vi "Core.vi"(8 "error in (no error)":errorcluster, 11 "Test 1 in":refnum<class "Test 1.lvclass">) -> (0 "error out":errorcluster, 3 "Actor out":refnum<class "Actor.lvclass">)   [LabVIEW 2020, in "Scratchpad.lvlib" / "Test 1.lvlib" / "Test 1.lvclass"]
uses:
  Test 1.lvclass
  Artifex/Actor/Actor.lvclass
panel:
  out "Chart":dbl(graph)
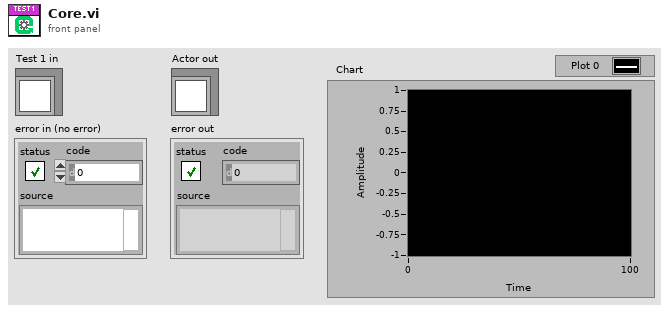
[diagram p1: front panel]
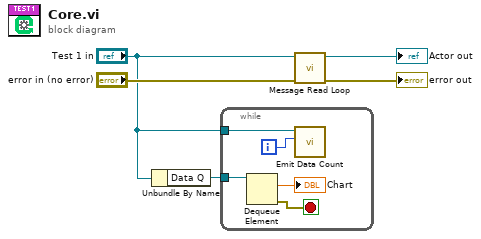
[diagram p0: block diagram]
diagram:
  n1 = Unbundle By Name("Test 1 in") -> ("Data Q"=w2:refnum<queue>)
  n2 = while {
    tunnel: w2 -> [w10]
    tunnel: "Test 1 in" -> [w7]
    i -> [w6]
    stop <- w8 stop-if-true
    n3 = Dequeue Element(queue=w10) -> (element=→"Chart":dbl, error out=w8:errorcluster)  [unwired: 2 in, 2 out]
    n4 = call "Emit Data Count.vi"("Data Count"=w6, "Test 1 API in"=w7) -> ()  [unwired: 8 in, 2 out]
  }
  n5 = call "Message Read Loop.vi"("error in (no error)"="error in (no error)", "Actor in"="Test 1 in") -> ("error out"=→"error out":errorcluster, "Actor out"=→"Actor out":refnum<class "Actor.lvclass">)  [unwired: 8 in]
